vi "Init_Instr.vi"(8 "error in (no error)":errorcluster caption="entrée d'erreur (pas d'erreur)", 11 "Class Instrument Multimeter en entrée":refnum<class "Class Instrument Multimeter.lvclass">) -> (0 "error out":errorcluster caption="sortie d'erreur", 3 "Class Instrument Multimeter en sortie":refnum<class "Class Instrument Multimeter.lvclass">)   [LabVIEW 2020, in "Library Instrument & Equipement.lvlib" / "Library Instruments.lvlib" / "Class Instrument Multimeter.lvclass"]
uses:
  Class Instrument Multimeter.lvclass
  Class Instrument Multimeter.lvclass/Class Instrument Multimeter.ctl
  Instrument (Default)/Class Instrument (Default).lvclass
  Multimeter/Multimeter (Default)/Class Multimeter (Default).lvclass
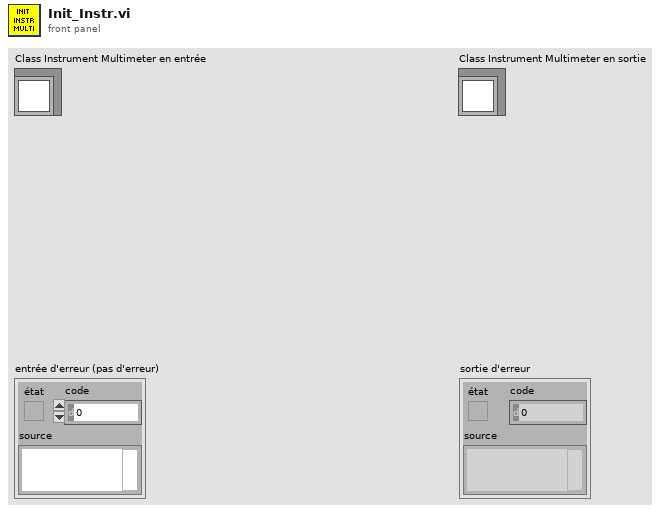
[diagram p1: front panel]
types:
  T1 = typedef "Library Commun.lvlib/Typedef Function.ctl" = enum16{"Voltmeter", "Ammeter", "Continuity", "Ohmmeter", "Frequencymeter"}
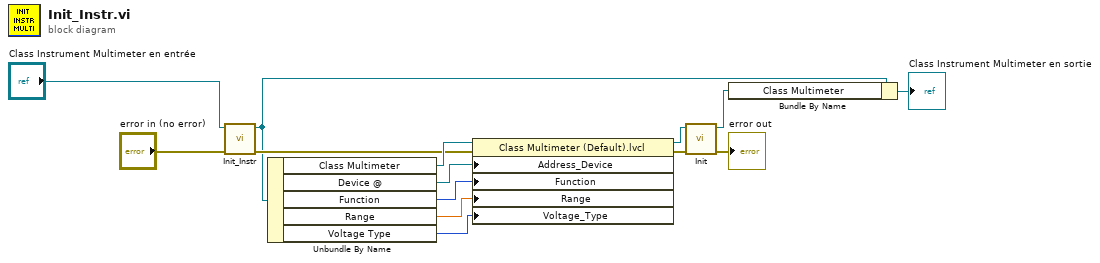
[diagram p0: block diagram]
diagram:
  n1 = call-parent "Init_Instr.vi"("error in (no error)"="error in (no error)", "Class Instrument (Default) en entrée"="Class Instrument Multimeter en entrée") -> ("error out"=w6:errorcluster, "Class Instrument (Default) en sortie"=w3:refnum<class "Class Instrument Multimeter.lvclass">)  [unwired: 8 in]
  n2 = Unbundle By Name(w3) -> ("Class Multimeter"=w11:refnum<class "Class Multimeter (Default).lvclass">, "Device @"=w10:refnum<visa-resource-name>, "Function"=w9:T1, "Range"=w8:dbl, "Voltage Type"=w7:enum16{"AC", "DC"})
  n3 = property class="Class Multimeter (Default).lvcl"(reference=w11, error in=w6, "Address_Device"=w10, "Function"=w9, "Range"=w8, "Voltage_Type"=w7) -> (reference out=w2:refnum<class "Class Multimeter (Default).lvclass">, error out=w5:errorcluster)
  n4 = call-dynamic "Init.vi"("error in (no error)"=w5, "Class Multimeter (Default) en entrée"=w2) -> ("error out"=→"error out":errorcluster, "Class Multimeter (Default) en sortie"=w1:refnum<class "Class Multimeter (Default).lvclass">)  [unwired: 8 in]
  n5 = Bundle By Name(cluster=w3, "Class Multimeter"=w1) -> (→"Class Instrument Multimeter en sortie":refnum<class "Class Instrument Multimeter.lvclass">)
